vi "Update Audio History.vi"(8 "error in (no error)":errorcluster, 9 "History Buffer Size (Samples) (44100)":i32=44100, 10 "Audio Data In":dbl[][](array[numeric]), 11 "Effect Interface in":refnum<class "Effect Interface.lvclass">) -> (0 "error out":errorcluster, 3 "Effect Interface out":refnum<class "Effect Interface.lvclass">)   [LabVIEW 2019, in "Effect Interface.lvlib" / "Effect Interface.lvclass"]
doc: "Updates the audio history buffer with new samples. If the history buffer doesn't exist, it is automatically created according to the sample size input.\n\nThe audio history buffer always has the oldest sample at index 0, and the latest sample at index (size - 1). As new samples are inserted into the history buffer, the buffer is rotated to maintain the oldest sample at index 0."
uses:
  Effect Interface.lvclass
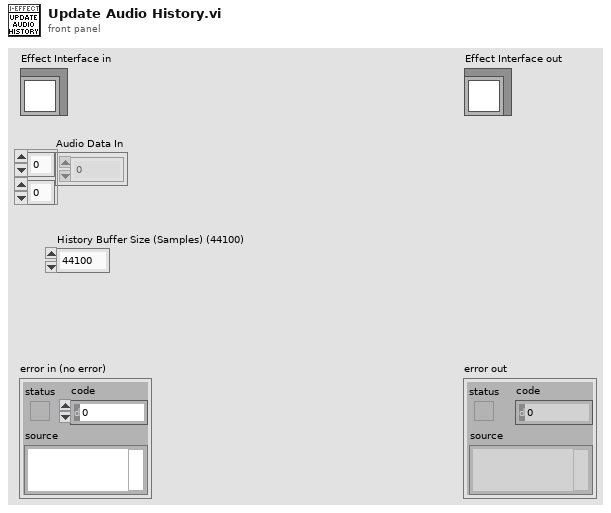
[diagram p1: front panel]
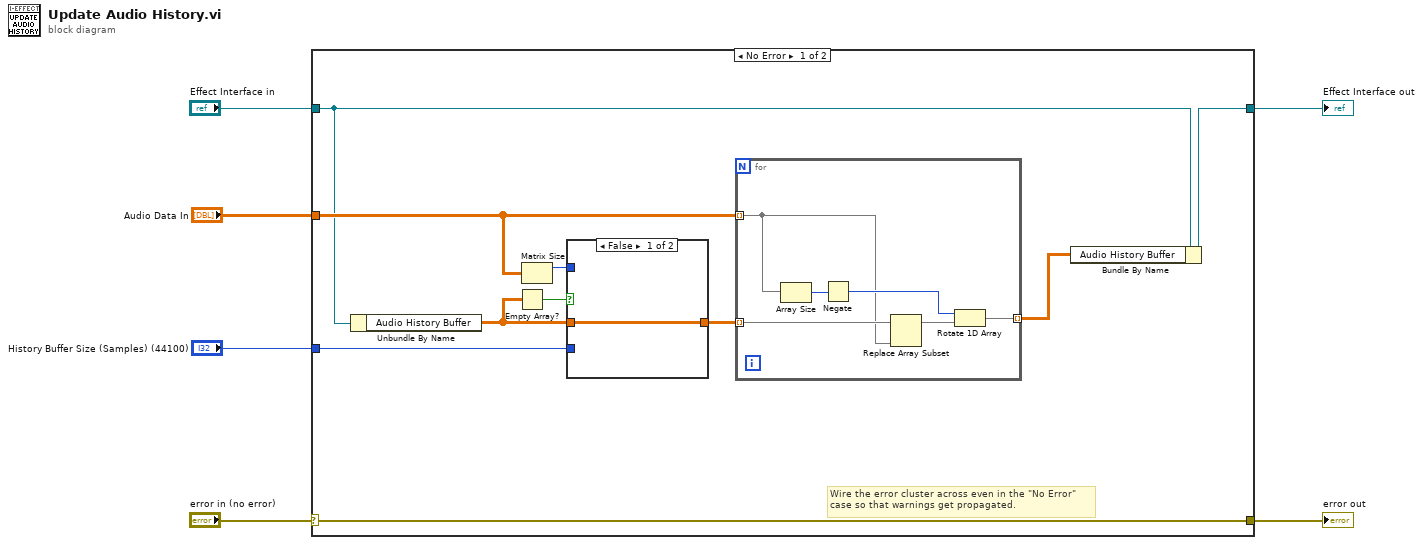
[diagram p0: block diagram]
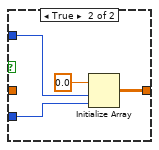
[diagram p2: hidden frame]
diagram:
  n1 = case shown="No Error" "error in (no error)" {
    selector: "error in (no error)" -> [w16 w29]
    tunnel: [w16 w29] -> w5
    tunnel: [w12 w28] -> w3
    tunnel: "Effect Interface in" -> [w11 w28]
    tunnel: "Audio Data In" -> [w13 _]
    tunnel: "History Buffer Size (Samples) (44100)" -> [w7 _]
    frame No Error {
      # "Wire the error cluster across even in the \"No Error\"\ncase so that warnings get propagated."
      n2 = Unbundle By Name(w11) -> ("Audio History Buffer"=w9:dbl[][])
      n3 = Empty Array?(array=w9) -> (empty?=w8:bool)
      n4 = Matrix Size(0:w13) -> (1:w14:i32)  [unwired: 1 out]
      n5 = case shown="False" w8 {
        tunnel: w9 -> [w23 _]
        tunnel: [w23 w25] -> w15
        tunnel: w14 -> [_ w27]
        tunnel: w7 -> [_ w24]
        frame False {
        }
        frame True {
          n6 = Initialize Array(0.0 ("element"), w27, w24) -> (w25:dbl[][])
        }
      }
      n7 = for {
        tunnel: w13 -> [w17] mode=indexing
        tunnel: w15 -> [w20] mode=indexing
        tunnel: [w18] -> w10 mode=indexing
        n8 = Array Size(array=w17) -> (size(s)=w22:i32)
        n9 = Negate(x=w22) -> (-x=w21:i32)
        n10 = Replace Array Subset(array=w20, new element=w17) -> (w19:dbl[])  [unwired: 1 in]
        n11 = Rotate 1D Array(1:w19, 2:w21) -> (0:w18:dbl[])
      }
      n12 = Bundle By Name(cluster=w11, "Audio History Buffer"=w10) -> (w12:refnum<class "Effect Interface.lvclass">)
    }
    frame Error {
    }
  }
  "error out" <- w5
  "Effect Interface out" <- w3
